vi "Read Pulse Configuration.vi"(8 "error in (no error)":errorcluster, 11 "Micron Optics Driver in":refnum<class "Micron Optics Driver.lvclass">) -> (0 "error out":errorcluster, 2 "Configuration":T1={"Post-trigger delay"=0.01, "Post-trigger duration"=0.1, "Rate"=1000000.0, "Ranges"=[10.0], "Re-name channels"=[], "Active channels"="0:1", "External clock"=FALSE} {"Rate" format="%#_8pHz"; "Post-trigger duration" format="%#_6ps"; "Post-trigger delay" format="%#_6ps"; "Ranges" format="%#_6pV"}, 3 "Micron Optics Driver out":refnum<class "Micron Optics Driver.lvclass">)   [LabVIEW 2024, in "Micron Optics Driver.lvclass"]
uses:
  Micron Optics Driver.lvclass
  Pulse Driver/Pusle Driver Configuration.ctl
  Micron Optics Driver.lvclass/Micron Optics Driver.ctl
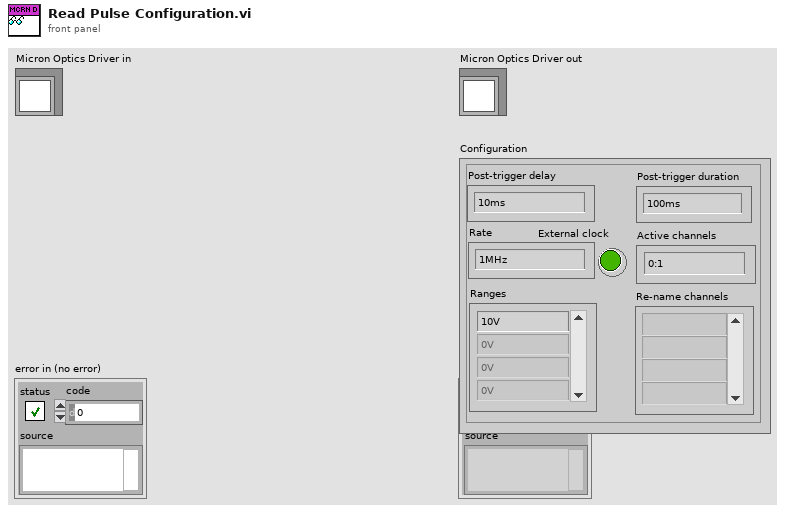
[diagram p1: front panel]
types:
  T1 = typedef "Pusle Driver Configuration.ctl" = cluster{"Post-trigger delay":dbl, "Post-trigger duration":dbl, "Rate":dbl, "Ranges":dbl[], "Re-name channels":string[], "Active channels":string, "External clock":bool}
  T2 = typedef "Micron optics didgitizer configuration.ctl" = cluster{"Post-trigger delay":dbl, "Post-trigger duration":dbl, "Rate":dbl, "Reference channel":i32, "Detection Setting IDs":u8[], "Stream and average":bool, "Address":string}
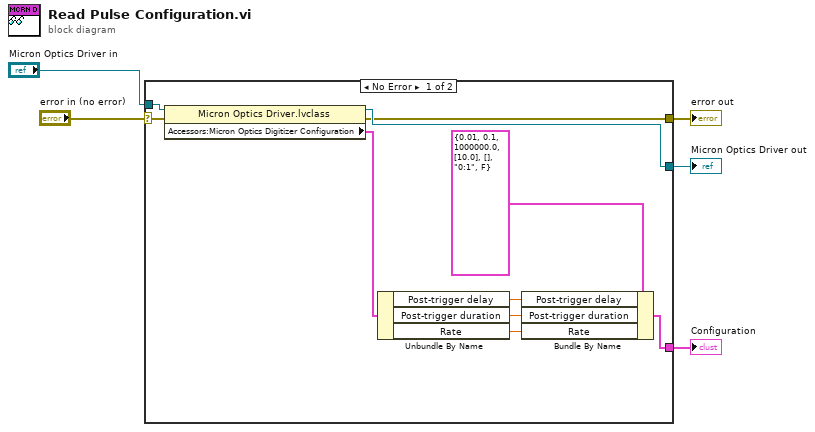
[diagram p0: block diagram]
diagram:
  n1 = case shown="No Error" "error in (no error)" {
    selector: "error in (no error)" -> [w7 w16]
    tunnel: [w8 w16] -> w4
    tunnel: [w9 w17] -> w2
    tunnel: "Micron Optics Driver in" -> [w10 w17]
    tunnel: [w6 _] -> w1
    frame No Error {
      n2 = property class="Micron Optics Driver.lvclass"(reference=w10, error in=w7) -> (reference out=w9:refnum<class "Micron Optics Driver.lvclass">, error out=w8:errorcluster, "Accessors:Micron Optics Digitizer Configuration"=w12:T2)
      n3 = Unbundle By Name(w12) -> ("Post-trigger delay"=w15:dbl, "Post-trigger duration"=w14:dbl, "Rate"=w13:dbl)
      n4 = Bundle By Name(cluster=T1 {"Post-trigger delay"=0.01, "Post-trigger duration"=0.1, "Rate"=1000000.0, "Ranges"=[10.0], "Re-name channels"=[], "Active channels"="0:1", "External clock"=FALSE} ("Pulse Driver Configuration"), "Post-trigger delay"=w15, "Post-trigger duration"=w14, "Rate"=w13) -> (w6:T1)
    }
    frame Error {
    }
  }
  "error out" <- w4
  "Micron Optics Driver out" <- w2
  "Configuration" <- w1
